vi "CliListBlocksOfType.vi"(0 "ref in":u64, 7 "BlockType":i32(ring)=65 items=["OB"=56, "DB"=65, "SDB"=66, "FC"=67, "SFC"=68, "FB"=69, "SFB"=70], 11 "error in (no error)":errorcluster) -> (4 "ref out":u64, 6 "Result":i32, 8 "BlockList":u16[](array[numeric]), 10 "ItemsCount":i32, 15 "error out":errorcluster)   [LabVIEW 2016, in "Snap7.lvlib"]
uses:
  Snap7.lvlib
  win32/lv_snap7.dll
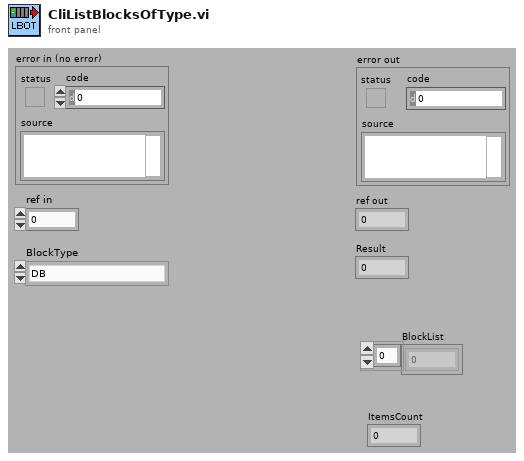
[diagram p1: front panel]
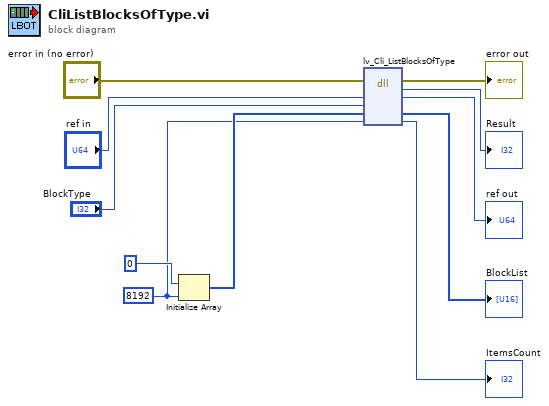
[diagram p0: block diagram]
diagram:
  w3 = 8192
  n1 = Initialize Array(u16 0, w3) -> (w4:u16[])
  n2 = dll-call lib="D:/maszup/svn/LineTraceSystem/SOFTWARE/sources/Drivers/PLC/Snap7/lib/win32/lv_snap7.dll" fn="lv_Cli_ListBlocksOfType"(error in="error in (no error)", "Client"="ref in", "BlockType"="BlockType", "pUsrData"=w4, "ItemsCount"=w3) -> (error out=→"error out":errorcluster, "return type"=→"Result":i32, "Client"=→"ref out":u64, "pUsrData"=→"BlockList":u16[], "ItemsCount"=→"ItemsCount":i32)  [unwired: 3 in, 1 out]
